vi "自适应屏幕分辨率测试.vi"() -> ()   [LabVIEW 2017]
panel:
  in  "退出":bool
  in  "自适应分辨率":bool
  in  "Multicolumn Listbox":i32(listbox)
  out "Waveform Chart":dbl(graph)
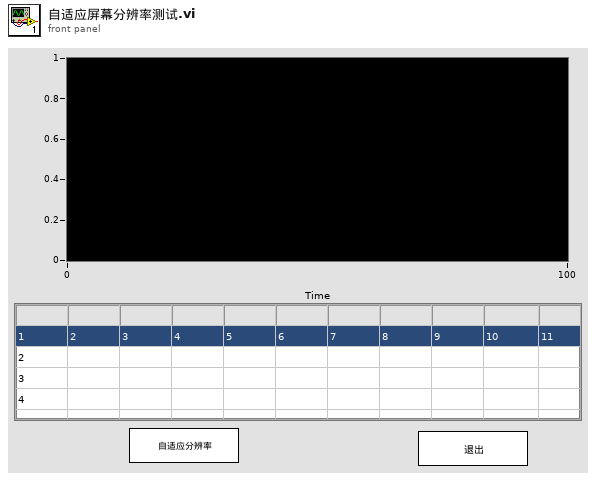
[diagram p1: front panel]
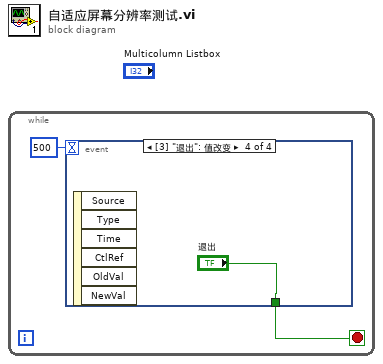
[diagram p0: block diagram]
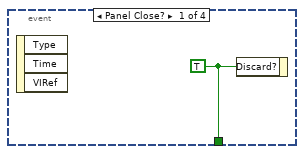
[diagram p2: hidden frame]
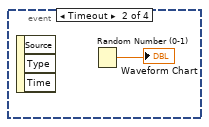
[diagram p3: hidden frame]
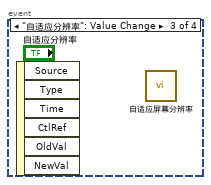
[diagram p4: hidden frame]
diagram:
  n1 = while {
    stop <- w2 stop-if-true
    n2 = event shown="[3] \"退出\": 值改变" {
      selector: _ -> [_ _ _ _]
      dyn-events: _ -> [_ _ _ _]
      timeout: 500 -> [_ _ _ _]
      tunnel: [w3 _ _ "退出"] -> w2
      event Panel Close? {
        w3 = TRUE ("Discard?")
        n3 = event-data() -> ()  [unwired: 1 in, 3 out]
        n4 = event-data("Discard?"=w3) -> ()  [unwired: 1 in, 1 out]
      }
      event Timeout {
        n5 = event-data() -> ()  [unwired: 1 in, 3 out]
        n6 = Random Number (0-1)() -> (number: 0 to 1=→"Waveform Chart":dbl)
      }
      event "自适应分辨率": Value Change {
        n7 = event-data() -> ()  [unwired: 1 in, 6 out]
        n8 = call "自适应屏幕分辨率.vi"() -> ()  [unwired: 16 in]
      }
      event "退出": Value Change {
        n9 = event-data() -> ()  [unwired: 1 in, 6 out]
      }
    }
  }
